vi "Desktop Main.vi"() -> ()   [LabVIEW 2013]
uses:
  SubVIs/Web Messaging API.lvlib
panel:
  out "Message List":T1(array[cluster])
  in  "stop":bool
  out "Error List from myRIO":T2(array[cluster])
  out "error out":errorcluster
  in  "Services Token":string
  # "This app demonstrates how to use the myRIO Web App messaging and monitoring web site\n-Get started by visiting https://myrio.niwsc.com and creating an account\n-On the myRIO Web App click 'My account' and then click 'Services token'\n-On the Services token tab click 'Generate new token'\n-Copy your new services token and paste it in this VI's Services Token control\n-Run the RT Main.vi on the myRIO\n-Run this VI and see  the messages and errors from the myRIO"
  # "The Services Token is generated on the myRIO Web App site\nVisit https://myrio.niwsc.com to get started"
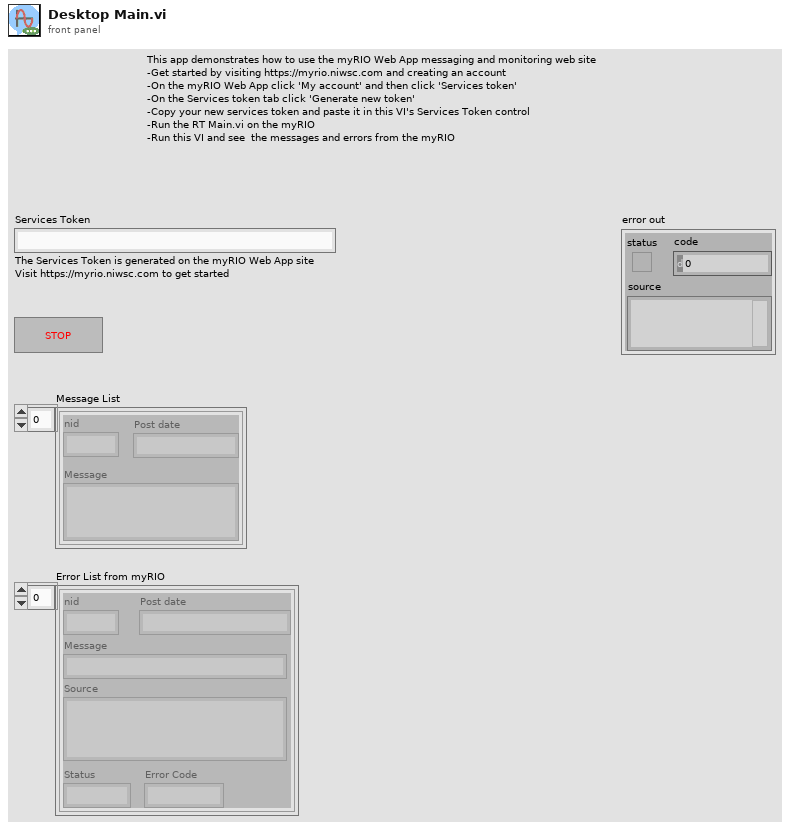
[diagram p1: front panel]
types:
  T1 = cluster{"nid":string, "Post date":string, "Message":string}[]
  T2 = cluster{"nid":string, "Post date":string, "Message":string, "Source":string, "Error Code":string, "Status":string}[]
  T3 = typedef "Web Messaging API.lvlib/Web Messaging Handle.ctl" = cluster{"Services token":string}
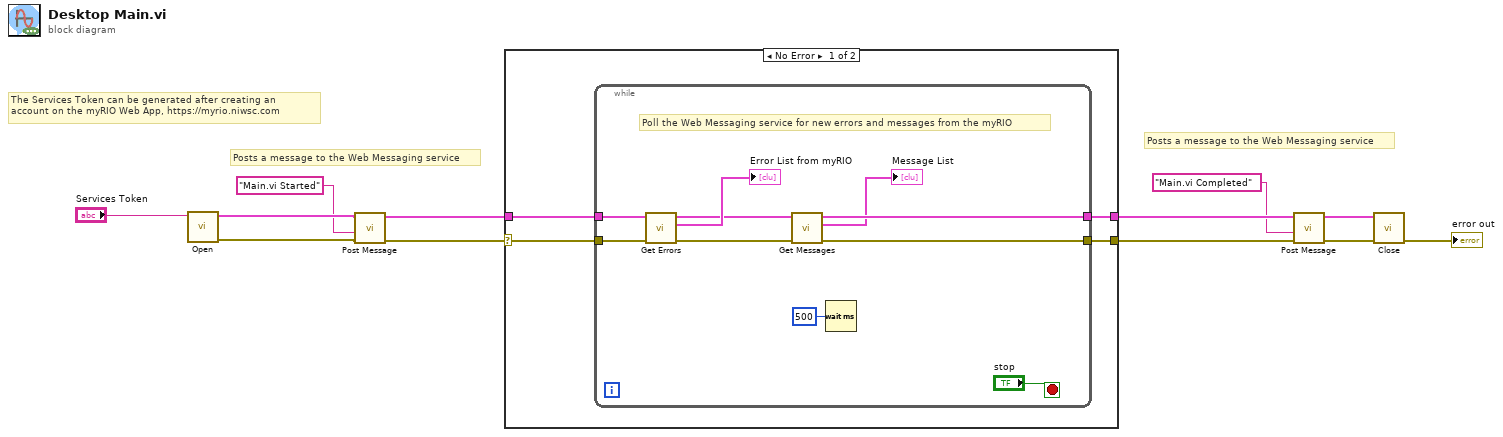
[diagram p0: block diagram]
diagram:
  # "Posts a message to the Web Messaging service"
  # "Posts a message to the Web Messaging service"
  # "The Services Token can be generated after creating an \naccount on the myRIO Web App, https://myrio.niwsc.com"
  n1 = call "Open.vi"("Services Token"="Services Token") -> ("error out"=w5:errorcluster, "Web App Handle"=w7:T3)  [unwired: 9 in]
  n2 = call "Post Message.vi"("error in (no error)"=w5, "message"="Main.vi Started", "Web App Handle In"=w7) -> ("error out"=w10:errorcluster, "Web App Handle Out"=w9:T3)  [unwired: 6 in, 1 out]
  n3 = case shown="No Error" w10 {
    selector: w10 -> [w14 w28]
    tunnel: [w13 w28] -> w11
    tunnel: w9 -> [w16 w27]
    tunnel: [w15 w27] -> w8
    frame No Error {
      n4 = while {
        tunnel: w16 -> [w25]
        tunnel: [w24] -> w15
        tunnel: w14 -> [w23]
        tunnel: [w22] -> w13
        stop <- "stop" stop-if-true
        # "Poll the Web Messaging service for new errors and messages from the myRIO"
        n5 = call "Get Errors.vi"("Web App Handle In"=w25, "error in"=w23) -> ("Web App Handle Out"=w18:T3, "Error List"=→"Error List from myRIO":T2, "error out"=w19:errorcluster)  [unwired: 6 in]
        n6 = call "Get Messages.vi"("Web App Handle In"=w18, "error in"=w19) -> ("Web App Handle Out"=w24:T3, "Message List"=→"Message List":T1, "error out"=w22:errorcluster)  [unwired: 6 in]
        n7 = Wait (ms)(milliseconds to wait=u32 500) -> ()  [unwired: 1 out]
      }
    }
    frame Error {
    }
  }
  n8 = call "Post Message.vi"("error in (no error)"=w11, "message"="Main.vi Completed", "Web App Handle In"=w8) -> ("error out"=w2:errorcluster, "Web App Handle Out"=w1:T3)  [unwired: 6 in, 1 out]
  n9 = call "Close.vi"("error in"=w2, "Web App Handle"=w1) -> ("error out"=→"error out":errorcluster)  [unwired: 9 in]
